vi "Walk (SubVI).vi"(6 "Boolean":bool, 7 "Reset To Cabin":bool, 9 "Y":i32, 10 "Array in":cluster{"X Cord":i32[], "Y Cord":i32[]}[](array[cluster]), 11 "X":i32) -> (3 "Array out":cluster{"Y":i32[], "\nX":i32[]}[](array[cluster]))   [LabVIEW 2021]
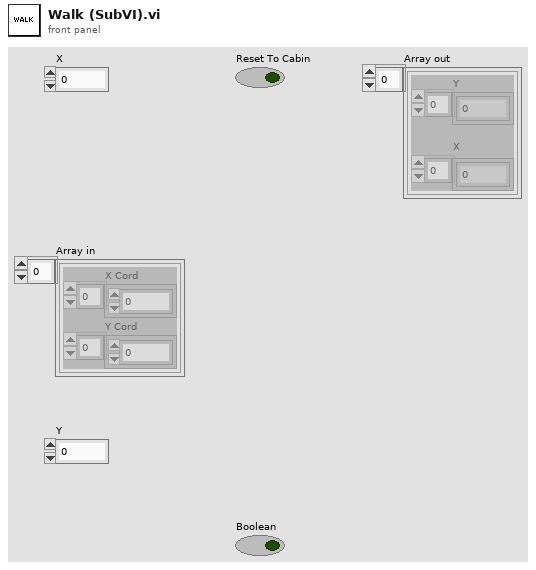
[diagram p1: front panel]
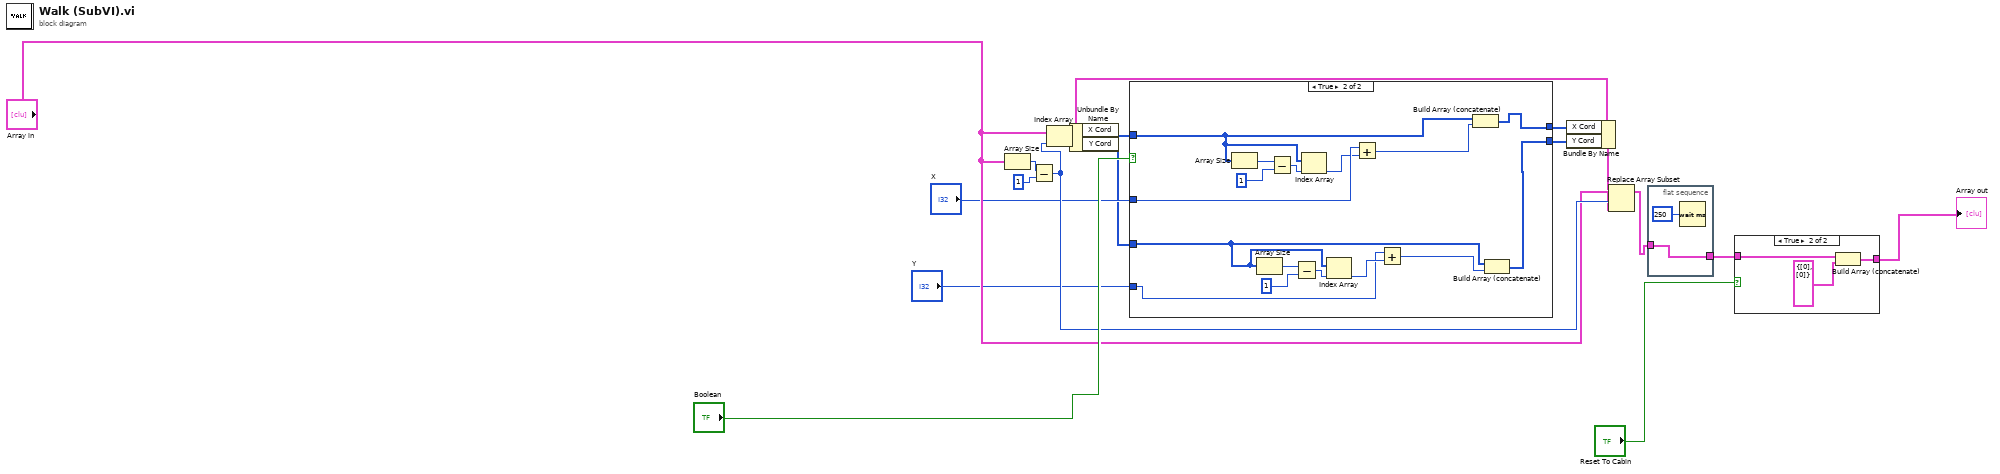
[diagram p0: block diagram]
diagram:
  n1 = Array Size(array="Array in") -> (size(s)=w14:i32)
  n2 = Subtract(x=w14, y=1) -> (x-y=w16:i32)
  n3 = Index Array(array="Array in", index=w16) -> (element=w11:cluster{"X Cord":i32[], "Y Cord":i32[]})
  n4 = Unbundle By Name(w11) -> ("X Cord"=w5:i32[], "Y Cord"=w6:i32[])
  n5 = case shown="True" "Boolean" {
    tunnel: w5 -> [w19 w30]
    tunnel: w6 -> [w18 w21]
    tunnel: [w19 w35] -> w7
    tunnel: [w18 w34] -> w8
    tunnel: "X" -> [_ w29]
    tunnel: "Y" -> [_ w22]
    frame False {
    }
    frame True {
      n6 = Array Size(array=w30) -> (size(s)=w32:i32)
      n7 = Array Size(array=w21) -> (size(s)=w25:i32)
      n8 = Subtract(x=w32, y=1) -> (x-y=w31:i32)
      n9 = Subtract(x=w25, y=1) -> (x-y=w24:i32)
      n10 = Index Array(array=w30, index=w31) -> (element=w28:i32)
      n11 = Index Array(array=w21, index=w24) -> (element=w23:i32)
      n12 = Add(x=w29, y=w28) -> (x+y=w27:i32)
      n13 = Add(x=w22, y=w23) -> (x+y=w20:i32)
      n14 = Build Array (concatenate)(w30, w27) -> (w35:i32[])
      n15 = Build Array (concatenate)(w21, w20) -> (w34:i32[])
    }
  }
  n16 = Bundle By Name(cluster=w11, "X Cord"=w7, "Y Cord"=w8) -> (w12:cluster{"X Cord":i32[], "Y Cord":i32[]})
  n17 = Replace Array Subset(array="Array in", new element=w12, index=w16) -> (w2:cluster{"X Cord":i32[], "Y Cord":i32[]}[])
  n18 = flat-sequence {
    tunnel: w2 -> [w37]
    tunnel: [w37] -> w1
    frame #0 {
      n19 = Wait (ms)(milliseconds to wait=u32 250) -> ()  [unwired: 1 out]
    }
  }
  n20 = case shown="True" "Reset To Cabin" {
    tunnel: w1 -> [w38 w40]
    tunnel: [w38 w41] -> w3
    frame False {
    }
    frame True {
      n21 = Build Array (concatenate)(w40, cluster{"Y":i32[], "\nX":i32[]} {"Y"=[0], "\nX"=[0]}) -> (w41:cluster{"Y":i32[], "\nX":i32[]}[])
    }
  }
  "Array out" <- w3
